vi "forchetta.vi"() -> ()   [LabVIEW 2020]
panel:
  out "error out":errorcluster
  in  "error in (no error)":errorcluster
  in  "Image Path":path
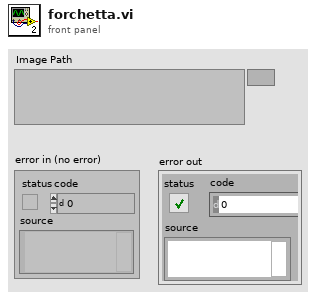
[diagram p1: front panel]
types:
  T1 = typedef "IMAQ Image.ctl" = refnum<image>
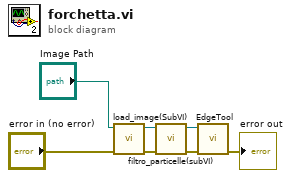
[diagram p0: block diagram]
diagram:
  n1 = call "load_image(SubVI).vi"("error in (no error)"="error in (no error)", "Image Path"="Image Path") -> ("error out"=w2:errorcluster, "Image GRAY"=w4:T1)  [unwired: 7 in, 1 out]
  n2 = call "filtro_particelle(subVI).vi"("error in (no error)"=w2, "Image Src"=w4) -> ("error out"=w1:errorcluster, "Image"=w3:T1)  [unwired: 8 in]
  n3 = call "EdgeTool.vi"("error in (no error)"=w1, "New Image"=w3) -> ("error out"=→"error out":errorcluster)  [unwired: 8 in, 1 out]
